vi "DDS9959 Set Amplitude.vi"(0 "VISA resource name":refnum<visa-resource-name>, 1 "ramp rate":u8 max=1, 5 "Set Amplitude Scale Factor":dbl format="%#_10g", 7 "Channel":u16=1 min=1 max=4, 9 "Amplitude Control Register":T1, 11 "error in (no error)":errorcluster) -> (4 "VISA resource name out":refnum<visa-resource-name>, 15 "error out":errorcluster)   [LabVIEW 2012]
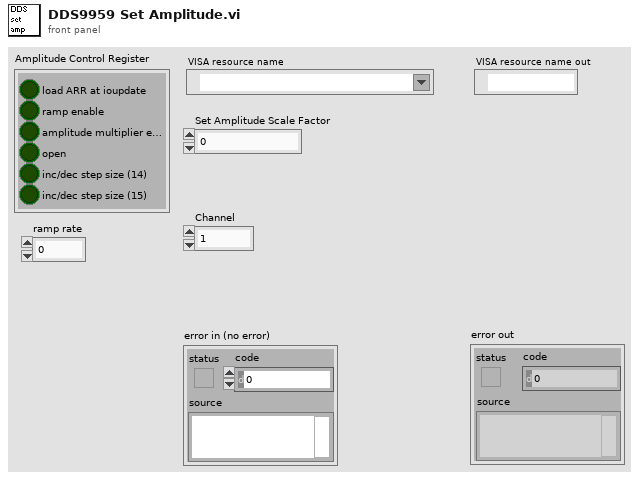
[diagram p1: front panel]
types:
  T1 = cluster{"load ARR at ioupdate":bool, "ramp enable":bool, "amplitude multiplier enable":bool, "open":bool, "inc/dec step size (14)":bool, "inc/dec step size (15)":bool}
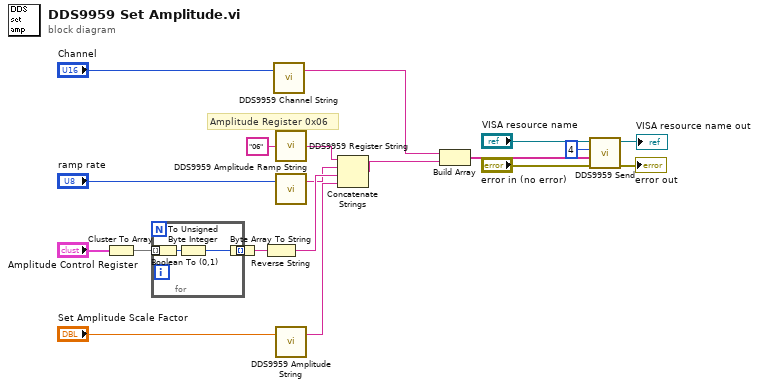
[diagram p0: block diagram]
diagram:
  # "Amplitude Register 0x06"
  n1 = Cluster To Array(cluster="Amplitude Control Register") -> (array=w13:bool[])
  n2 = for {
    tunnel: w13 -> [w21] mode=indexing
    tunnel: [w22] -> w15 mode=indexing
    n3 = Boolean To (0,1)(Boolean=w21) -> (0, 1=w23:i16)
    n4 = To Unsigned Byte Integer(number=w23) -> (unsigned 8bit integer=w22:u8)
  }
  n5 = Byte Array To String(unsigned byte array=w15) -> (string=w14:string)
  n6 = Reverse String(1:w14) -> (0:w10:string)
  n7 = call "DDS9959 Channel String.vi"("Channel"="Channel") -> ("String"=w5:string)  [unwired: 2 in]
  n8 = call "DDS9959 Register String.vi"("register"="06") -> ("output"=w11:string)
  n9 = call "DDS9959 Amplitude Ramp String.vi"("Ramp Step (us)"="ramp rate") -> ("String"=w3:string)  [unwired: 2 in]
  n10 = call "DDS9959 Amplitude String.vi"("Set Amplitude Scale Factor"="Set Amplitude Scale Factor") -> ("String"=w9:string)  [unwired: 2 in]
  n11 = Concatenate Strings(w11, w3, w10, w9) -> (w18:string)
  n12 = Build Array(w5, w18) -> (w20:string[])
  n13 = call "DDS9959 Send.vi"("error in (no error)"="error in (no error)", "Output Array"=w20, "USB Out Endpoint"=i16 4, "VISA resource name"="VISA resource name") -> ("error out"=→"error out":errorcluster, "VISA resource name"=→"VISA resource name out":refnum<visa-resource-name>)  [unwired: 6 in]
